vi "Timeout Phase.vi"(8 "error in (no error)":errorcluster, 11 "Programming Logicv2 in":refnum<class "Programming Logicv2.lvclass">) -> (0 "error out":errorcluster, 1 "Boolean":bool, 3 "Programming Logicv2 out":refnum<class "Programming Logicv2.lvclass">, 9 "Timer":u16, 10 "Temperature":u16)   [LabVIEW 2014, in "Main Libraryv2.lvlib" / "Programming Logicv2.lvclass"]
uses:
  Programming Logicv2.lvclass
  Control/Main Libraryv2.lvlib
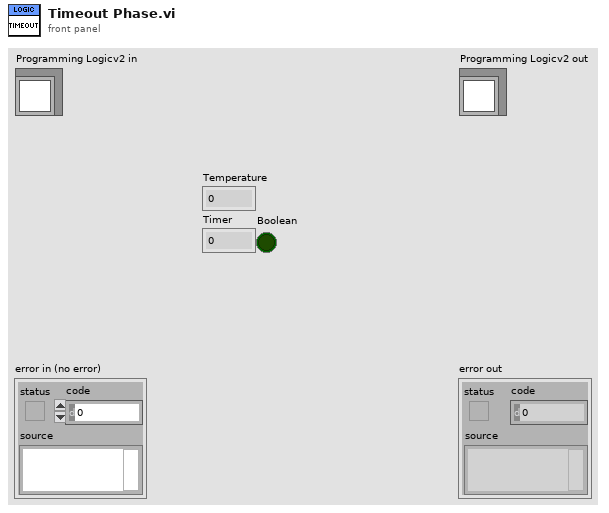
[diagram p1: front panel]
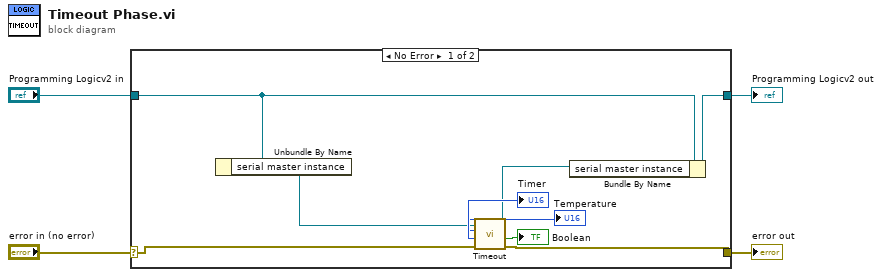
[diagram p0: block diagram]
diagram:
  n1 = case shown="No Error" "error in (no error)" {
    selector: "error in (no error)" -> [w10 w15]
    tunnel: [w9 w15] -> w3
    tunnel: [w7 w14] -> w1
    tunnel: "Programming Logicv2 in" -> [w6 w14]
    frame No Error {
      n2 = Unbundle By Name(w6) -> ("serial master instance"=w5:refnum<class "Modbus Master.lvclass">)
      n3 = call "Timeout.vi"("error in"=w10, "Modbus master in"=w5) -> ("error out"=w9:errorcluster, "Boolean"=→"Boolean":bool, "Modbus master out"=w8:refnum<class "Modbus Master.lvclass">, "Timer"=→"Timer":u16, "Temperature"=→"Temperature":u16)  [unwired: 5 in]
      n4 = Bundle By Name(cluster=w6, "serial master instance"=w8) -> (w7:refnum<class "Programming Logicv2.lvclass">)
    }
    frame Error {
    }
  }
  "error out" <- w3
  "Programming Logicv2 out" <- w1
